vi "FGVPartB.vi"() -> ()   [LabVIEW 2014]
panel:
  out "Count":i32
  in  "stop":bool
  out "NumericOut":i32
  # "PartB"
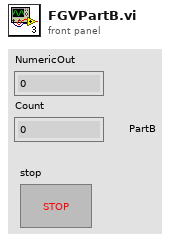
[diagram p1: front panel]
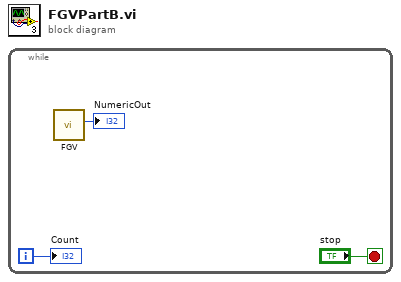
[diagram p0: block diagram]
diagram:
  n1 = while {
    i -> [w1]
    stop <- "stop" stop-if-true
    n2 = call "FGV.vi"() -> ("NumericOut"=→"NumericOut":i32)  [unwired: 11 in]
    "Count" <- w1
  }
